vi "Ini file-Open.vi"(8 "Error In":errorcluster, 11 "Which file?":T1=enum."Setup.ini") -> (0 "error out":errorcluster, 1 "file created?":bool, 2 "Path Out":path, 3 "User profile ini file ref":T2)   [LabVIEW 2020]
uses:
  <vilib>/Utility/config.llb/Config Data RefNum.ctl
  Typedefs/Which path.ctl
  <vilib>/Utility/config.llb/NI_LVConfig.lvlib
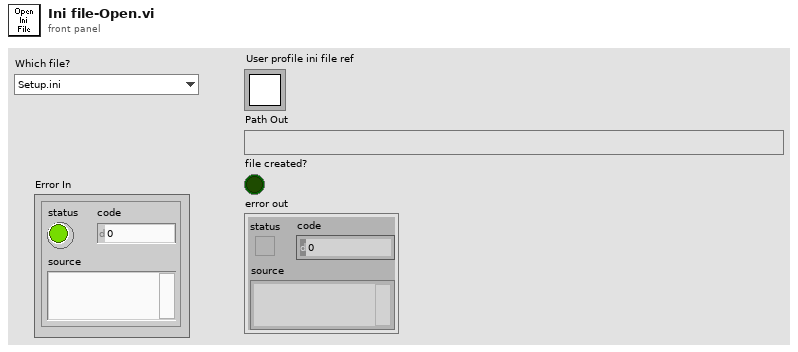
[diagram p1: front panel]
types:
  T1 = typedef "Which path.ctl" = enum16{"Configuration Files", "Calibration Files", "Images", "Setup.ini", "Loaded User profile.ini", "User's-Previous session.ini", "New user profile.ini", "Selected User profile.ini", "User profiles folder", "Power meter scaling.txt", "FOV Cal.ini", "Calibration.ini"}
  T2 = typedef "NI_LVConfig.lvlib/Config Data RefNum.ctl" = refnum<k1>
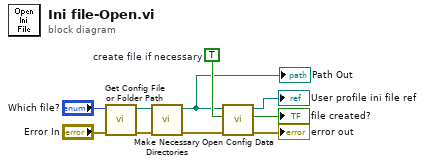
[diagram p0: block diagram]
diagram:
  w9 = TRUE  # create file if necessary
  n1 = call "Get Config File or Folder Path.vi"("Error In"="Error In", "Which file or folder?"="Which file?") -> ("Error Out"=w2:errorcluster, "File Path"=w4:path)  [unwired: 7 in, 1 out]
  n2 = call <userlib>:"Make Necessary Directories.vi"("error in"=w2, "Path"=w4) -> ("error out"=w10:errorcluster, "Duplicated path"=w3:path)  [unwired: 8 in]
  "Path Out" <- w3
  n3 = call <vilib>:"Open Config Data.vi"("error in (no error)"=w10, "create file if necessary (T)"=w9, "configuration file path"=w3) -> ("error out"=→"error out":errorcluster, "file created?"=→"file created?":bool, "refnum"=→"User profile ini file ref":T2)  [unwired: 6 in]
